vi "Store CRD Data.vi"(8 "error in":errorcluster, 11 "Controller in":refnum<class "Controller.lvclass">) -> (0 "error out":errorcluster, 3 "Controller out":refnum<class "Controller.lvclass">)   [LabVIEW 2014, in "Controller.lvlib" / "Controller.lvclass"]
uses:
  Controller.lvclass
  Controls/eMap.ctl
  <vilib>/ActorFramework/Message Enqueuer/Message Enqueuer.lvclass
  Instr Actor/Messages/Update Housekeeping/Update Housekeeping MSG.lvclass
  Controller.lvclass/Controller.ctl
  Instr Actor/Messages/Update Housekeeping/Update Housekeeping MSG.lvclass/Update Housekeeping MSG.ctl
  <vilib>/ActorFramework/Message Enqueuer/Message Enqueuer.lvclass/Message Enqueuer.ctl
  <vilib>/ActorFramework/Message Priority Queue/Priority Enqueue.vi
panel:
  out "DataOut":T1(array[cluster])
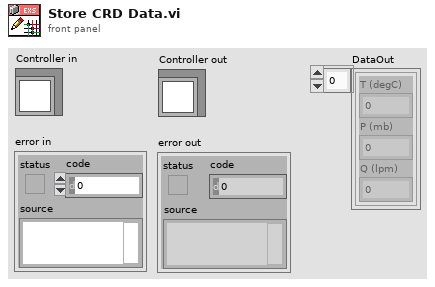
[diagram p1: front panel]
types:
  T1 = cluster{"T (degC)":dbl, "P (mb)":dbl, "Q (lpm)":dbl}[]
  T2 = cluster{"T (degC)":dbl, "P (mb)":dbl, "Q (lpm)":dbl}
  T3 = typedef "Controller.lvlib/Controller.lvclass/eMap.ctl" = cluster{"Enqueuer":refnum<class "Message Enqueuer.lvclass">, "Active":bool}
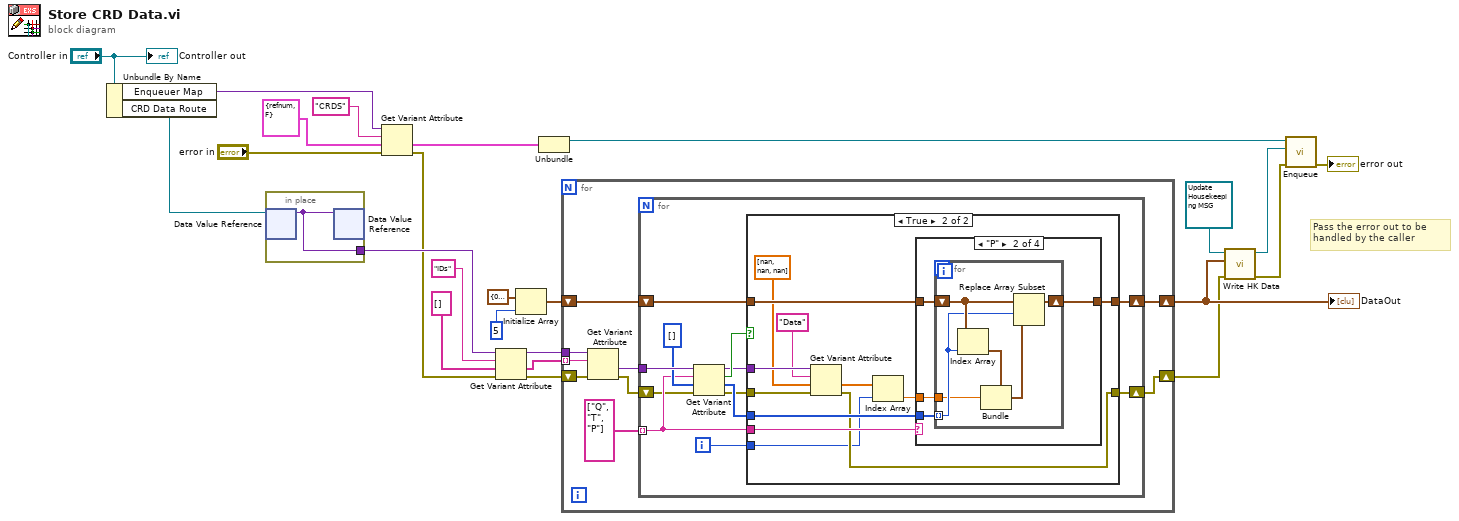
[diagram p0: block diagram]
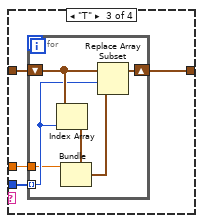
[diagram p4: hidden frame]
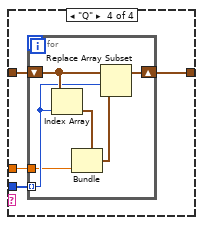
[diagram p5: hidden frame]
diagram:
  # "Pass the error out to be handled by the caller"
  n1 = Unbundle By Name("Controller in") -> ("Enqueuer Map"=w4:variant, "CRD Data Route"=w20:refnum<data-value>)
  n2 = in-place {
    in-place-border: [w25] -> w19
    n3 = in-place-dvr #1(w20) -> (w25:variant)  [unwired: 1 out]
    n4 = in-place-dvr #1(w25) -> ()  [unwired: 2 out]
  }
  n5 = Get Variant Attribute(Variant=w4, name="CRDS", default value (empty Variant)=T3 {"Enqueuer"=refnum, "Active"=FALSE} ("eMap"), error in="error in") -> (value=w21:T3, error out=w10:errorcluster)  [unwired: 2 out]
  n6 = Get Variant Attribute(Variant=w19, name="IDs", default value (empty Variant)=string[] [], error in=w10) -> (duplicate Variant=w15:variant, value=w16:string[], error out=w9:errorcluster)  [unwired: 1 out]
  n7 = Initialize Array(T2 {"T (degC)"=0.0, "P (mb)"=0.0, "Q (lpm)"=0.0} ("HK Data"), 5 ("dimension size")) -> (w12:T1)
  n8 = Unbundle(w21) -> ("Enqueuer"=w8:refnum<class "Message Enqueuer.lvclass">)  [unwired: 1 out]
  n9 = for {
    tunnel: w16 -> [w33] mode=indexing
    tunnel: w15 -> [w34]
    shift-right: [w30] -> w6
    shift-left: w12 -> [w31]
    shift-right: [w26] -> w3
    shift-left: w9 -> [w28]
    n10 = Get Variant Attribute(Variant=w34, name=w33, error in=w28) -> (value=w32:variant, error out=w27:errorcluster)  [unwired: 1 in, 2 out]
    n11 = for {
      tunnel: w32 -> [w46]
      shift-right: [w40] -> w30
      shift-left: w31 -> [w41]
      tunnel: string[] ["Q", "T", "P"] -> [w39] mode=indexing
      shift-right: [w36] -> w26
      shift-left: w27 -> [w38]
      i -> [w35]
      n12 = Get Variant Attribute(Variant=w46, name=w39, default value (empty Variant)=i32[] [], error in=w38) -> (duplicate Variant=w43:variant, found=w44:bool, value=w42:i32[], error out=w37:errorcluster)
      n13 = case shown="True" w44 {
        tunnel: w43 -> [_ w60]
        tunnel: w42 -> [_ w55]
        tunnel: w41 -> [w48 w57]
        tunnel: [w48 w56] -> w40
        tunnel: w39 -> [_ w58]
        tunnel: w37 -> [w47 w54]
        tunnel: [w47 w53] -> w36
        tunnel: w35 -> [_ w51]
        frame False {
        }
        frame True {
          n14 = Get Variant Attribute(Variant=w60, name="Data", default value (empty Variant)=dbl[] [nan, nan, nan], error in=w54) -> (value=w49:dbl[], error out=w53:errorcluster)  [unwired: 2 out]
          n15 = Index Array(array=w49, index=w51) -> (element=w50:dbl)
          n16 = case shown="\"P\"" w58 {
            tunnel: w57 -> [w61 w65 w75 w85]
            tunnel: [w61 w64 w74 w84] -> w56
            tunnel: w55 -> [_ w63 w72 w82]
            tunnel: w50 -> [_ w62 w73 w83]
            frame "NOOP", Default {
            }
            frame "P" {
              n17 = for {
                shift-right: [w67] -> w64
                shift-left: w65 -> [w71]
                tunnel: w63 -> [w70] mode=indexing
                tunnel: w62 -> [w68]
                n18 = Index Array(array=w71, index=w70) -> (element=w69:T2)
                n19 = Bundle(cluster=w69, "P (mb)"=w68) -> (w66:T2)  [unwired: 2 in]
                n20 = Replace Array Subset(array=w71, new element=w66, index=w70) -> (w67:T1)
              }
            }
            frame "T" {
              n21 = for {
                shift-right: [w78] -> w74
                shift-left: w75 -> [w81]
                tunnel: w72 -> [w80] mode=indexing
                tunnel: w73 -> [w77]
                n22 = Index Array(array=w81, index=w80) -> (element=w79:T2)
                n23 = Bundle(cluster=w79, "T (degC)"=w77) -> (w76:T2)  [unwired: 2 in]
                n24 = Replace Array Subset(array=w81, new element=w76, index=w80) -> (w78:T1)
              }
            }
            frame "Q" {
              n25 = for {
                shift-right: [w88] -> w84
                shift-left: w85 -> [w91]
                tunnel: w82 -> [w90] mode=indexing
                tunnel: w83 -> [w86]
                n26 = Index Array(array=w91, index=w90) -> (element=w89:T2)
                n27 = Bundle(cluster=w89, "Q (lpm)"=w86) -> (w87:T2)  [unwired: 2 in]
                n28 = Replace Array Subset(array=w91, new element=w87, index=w90) -> (w88:T1)
              }
            }
          }
        }
      }
    }
  }
  "DataOut" <- w6
  n29 = call "Write HK Data.vi"("error in (no error)"=w3, "HK Data"=w6, "Update Housekeeping MSG in"=refnum<class "Update Housekeeping MSG.lvclass"> refnum ("Instrument Lib:T_P MSG")) -> ("error out"=w2:errorcluster, "Update Housekeeping MSG out"=w5:refnum<class "Update Housekeeping MSG.lvclass">)  [unwired: 7 in]
  n30 = call <vilib>:"Enqueue.vi"("error in (no error)"=w2, "Message"=w5, "Message Enqueuer in"=w8) -> ("error out"=→"error out":errorcluster)  [unwired: 7 in, 1 out]
  "Controller out" <- "Controller in"
